vi "LogMultiStringEvent(Caller).vi"(8 "Error In":errorcluster, 10 "Data":variant[](array[variant]), 11 "Fields":string[](array[string])) -> (0 "Error Out":errorcluster)   [LabVIEW 2019, in "EventLogger.lvlib"]
uses:
  EventLogger.lvlib
  Enum - Message.ctl
  <vilib>/Utility/Data Type/NI_Data Type.lvlib
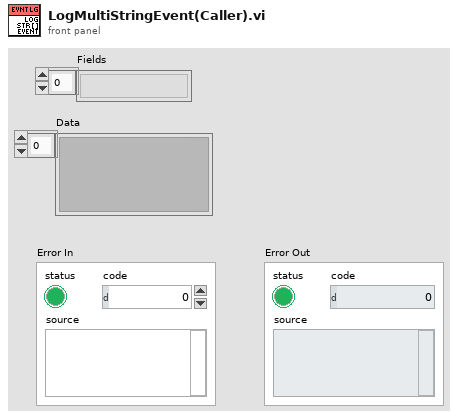
[diagram p1: front panel]
types:
  T1 = typedef "EventLogger.lvlib/Enum - Message.ctl" = enum16{"Initialize", "Idle", "CreateLog", "LogStrEvent", "LogErrorEvent", "LogVICall", "Error", "Exit"}
  T2 = typedef "NI_Data Type.lvlib/Data Type.ctl" = enum8{"Invalid Type", "Void", "I8", "I16", "I32", "I64", "U8", "U16", "U32", "U64", "Single Float", "Double Float", "Extended Float", "Single Complex", "Double Complex", "Extended Complex", "Enum U8", "Enum U16", "Enum U32", "Enum U64", "Single Float With Unit", "Double Float With Unit", "Extended Float With Unit", "Single Complex with Unit", "Double Complex with Unit", "Extended Complex with Unit", "Boolean", "String", "Path", "Picture", "Tag", "Array", "Cluster", "Variant", "LV Variant", "Waveform", "Timestamp", "Digital Waveform", "Digital Data", "ExpressData", "Refnum", "External Data", "VI", "Poly VI", "LabVIEW Class Instance", "Fixed Point", "Set Collection", "Map Collection"}
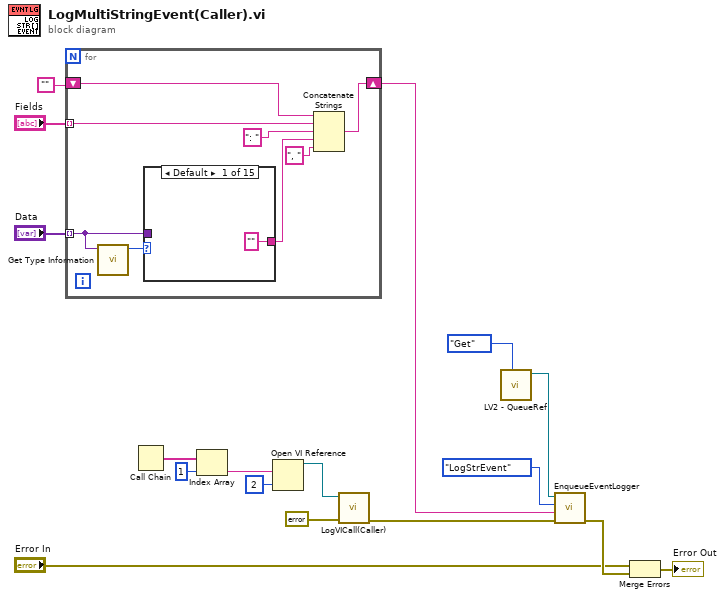
[diagram p0: block diagram]
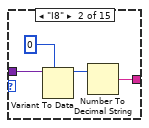
[diagram p2: hidden frame]
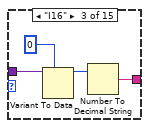
[diagram p3: hidden frame]
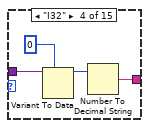
[diagram p4: hidden frame]
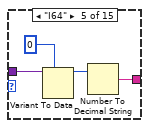
[diagram p5: hidden frame]
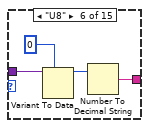
[diagram p6: hidden frame]
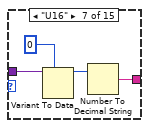
[diagram p7: hidden frame]
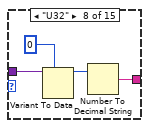
[diagram p8: hidden frame]
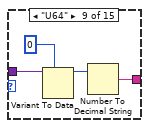
[diagram p9: hidden frame]
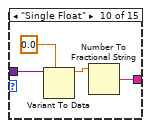
[diagram p10: hidden frame]
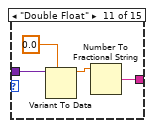
[diagram p11: hidden frame]
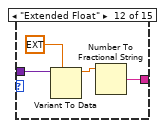
[diagram p12: hidden frame]
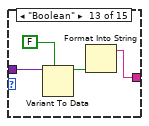
[diagram p13: hidden frame]
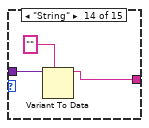
[diagram p14: hidden frame]
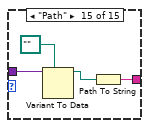
[diagram p15: hidden frame]
diagram:
  n1 = for {
    tunnel: "Fields" -> [w25] mode=indexing
    tunnel: "Data" -> [w22] mode=indexing
    shift-right: [w20] -> w1
    shift-left: "" -> [w19]
    n2 = call <vilib>:"Get Type Information.vi"("variant"=w22) -> ("type"=w23:T2)  [unwired: 6 in, 4 out]
    n3 = case shown="Default" w23 {
      tunnel: w22 -> [_ w29 w33 w37 w41 w45 w49 w53 w57 w61 w65 w69 w73 w76 w80]
      tunnel: ["" w27 w31 w35 w39 w43 w47 w51 w55 w59 w63 w67 w71 w75 w78] -> w21
      frame Default {
      }
      frame "I8" {
        n4 = Variant To Data(type=i8 0, Variant=w29) -> (data=w28:i8)  [unwired: 1 in, 1 out]
        n5 = Number To Decimal String(number=w28) -> (decimal integer string=w27:string)  [unwired: 1 in]
      }
      frame "I16" {
        n6 = Variant To Data(type=i16 0, Variant=w33) -> (data=w32:i16)  [unwired: 1 in, 1 out]
        n7 = Number To Decimal String(number=w32) -> (decimal integer string=w31:string)  [unwired: 1 in]
      }
      frame "I32" {
        n8 = Variant To Data(type=0, Variant=w37) -> (data=w36:i32)  [unwired: 1 in, 1 out]
        n9 = Number To Decimal String(number=w36) -> (decimal integer string=w35:string)  [unwired: 1 in]
      }
      frame "I64" {
        n10 = Variant To Data(type=i64 0, Variant=w41) -> (data=w40:i64)  [unwired: 1 in, 1 out]
        n11 = Number To Decimal String(number=w40) -> (decimal integer string=w39:string)  [unwired: 1 in]
      }
      frame "U8" {
        n12 = Variant To Data(type=u8 0, Variant=w45) -> (data=w44:u8)  [unwired: 1 in, 1 out]
        n13 = Number To Decimal String(number=w44) -> (decimal integer string=w43:string)  [unwired: 1 in]
      }
      frame "U16" {
        n14 = Variant To Data(type=u16 0, Variant=w49) -> (data=w48:u16)  [unwired: 1 in, 1 out]
        n15 = Number To Decimal String(number=w48) -> (decimal integer string=w47:string)  [unwired: 1 in]
      }
      frame "U32" {
        n16 = Variant To Data(type=u32 0, Variant=w53) -> (data=w52:u32)  [unwired: 1 in, 1 out]
        n17 = Number To Decimal String(number=w52) -> (decimal integer string=w51:string)  [unwired: 1 in]
      }
      frame "U64" {
        n18 = Variant To Data(type=u64 0, Variant=w57) -> (data=w56:u64)  [unwired: 1 in, 1 out]
        n19 = Number To Decimal String(number=w56) -> (decimal integer string=w55:string)  [unwired: 1 in]
      }
      frame "Single Float" {
        n20 = Variant To Data(type=sgl 0.0, Variant=w61) -> (data=w60:sgl)  [unwired: 1 in, 1 out]
        n21 = Number To Fractional String(number=w60) -> (F-format string=w59:string)  [unwired: 3 in]
      }
      frame "Double Float" {
        n22 = Variant To Data(type=0.0, Variant=w65) -> (data=w64:dbl)  [unwired: 1 in, 1 out]
        n23 = Number To Fractional String(number=w64) -> (F-format string=w63:string)  [unwired: 3 in]
      }
      frame "Extended Float" {
        n24 = Variant To Data(type=ext 0.0, Variant=w69) -> (data=w68:ext)  [unwired: 1 in, 1 out]
        n25 = Number To Fractional String(number=w68) -> (F-format string=w67:string)  [unwired: 3 in]
      }
      frame "Boolean" {
        n26 = Variant To Data(type=FALSE, Variant=w73) -> (data=w72:bool)  [unwired: 1 in, 1 out]
        n27 = Format Into String(w72) -> (resulting string=w71:string)  [unwired: 3 in, 1 out]
      }
      frame "String" {
        n28 = Variant To Data(type="", Variant=w76) -> (data=w75:string)  [unwired: 1 in, 1 out]
      }
      frame "Path" {
        n29 = Variant To Data(type=path "", Variant=w80) -> (data=w79:path)  [unwired: 1 in, 1 out]
        n30 = Path To String(path=w79) -> (string=w78:string)
      }
    }
    n31 = Concatenate Strings(w19, w25, ": " ("string"), w21, ", ") -> (w20:string)
  }
  n32 = Call Chain() -> (call chain=w12:string[])
  n33 = Index Array(array=w12, index=1) -> (element=w10:string)
  n34 = Open VI Reference(vi path=w10, options=2) -> (vi reference=w8:refnum<vi>)  [unwired: 4 in, 1 out]
  n35 = call "LogVICall(Caller).vi"("Error In"=errorcluster {"status"=FALSE, "code"=0, "source"=""}, "Caller VI"=w8) -> ("Error Out"=w13:errorcluster)  [unwired: 9 in]
  n36 = call "LV2 - QueueRef.vi"("Action"=enum16{"Set", "Get"}."Get") -> ("EventLoggerQueue out"=w15:refnum<queue>)  [unwired: 10 in]
  n37 = call "EnqueueEventLogger.vi"("Error In"=w13, "Data"=w1, "Message"=Enum_-_Message."LogStrEvent", "EventLoggerQueue"=w15) -> ("Error Out"=w16:errorcluster)  [unwired: 6 in, 1 out]
  n38 = Merge Errors("Error In", w16) -> (→"Error Out":errorcluster)
